vi "Zaber_Init.vi"() -> (0 "Assignment":cluster{"Microstep Size":dbl, "Device":string}[](array[cluster]), 1 "Axes Ass":bool, 2 "VISA resource name out":refnum<visa-resource-name>)   [LabVIEW 2015]
uses:
  <vilib>/Utility/file.llb/Read Delimited Spreadsheet (string).vi
  Zaber A Series/Zaber A Series.lvlib
panel:
  out "Microsteps":dbl[](array[numeric])
  out "error out":errorcluster
  out "Dev Numbers":string[](array[string])
  in  "Z":u16(ring) caption="Z (transverse)" items=["01", "02", "03"]
  in  "Y":u16(ring) caption="Y (vertical)" items=["01", "02", "03"]
  in  "X":u16(ring) caption="X (horizontal)" items=["01", "02", "03"]
  in  "Ass Axes":bool
  in  "Quit":bool
  in  "VISA resource name":refnum<visa-resource-name>
  out "Lookup file not found":bool
  in  "connect":bool
  out "Hardware Detected:":T1(array[cluster])
  out "Init Failed":bool
  # "Device Number & Axis"
  # "Model Name"
  # "Motion Type"
  # "Microstep"
  # "Assignment"
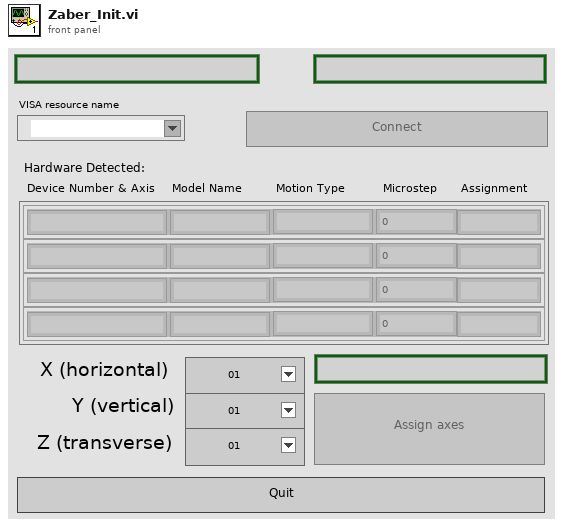
[diagram p1: front panel]
types:
  T1 = cluster{"Device Number & Axis":string, "Model Name":string, "Motion Type":string, "Microstep Size":dbl, "Assignment":string}[]
  T2 = enum8{"Enabled", "Disabled", "Disabled and Grayed Out"}
  T3 = cluster{"Device Number & Axis":string, "Model Name":string, "Motion Type":string, "Microstep Size":dbl, "Assignment":string}
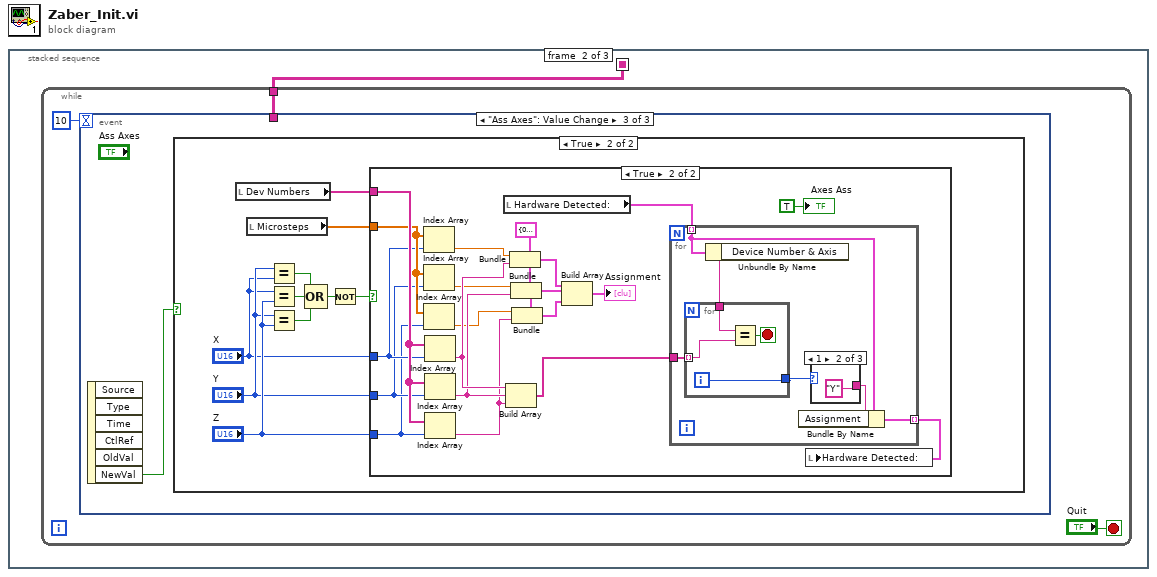
[diagram p0: block diagram]
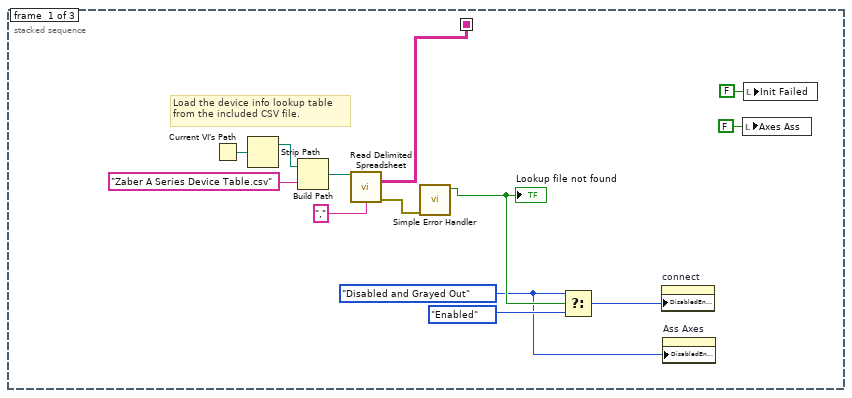
[diagram p2: hidden frame]
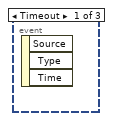
[diagram p3: hidden frame]
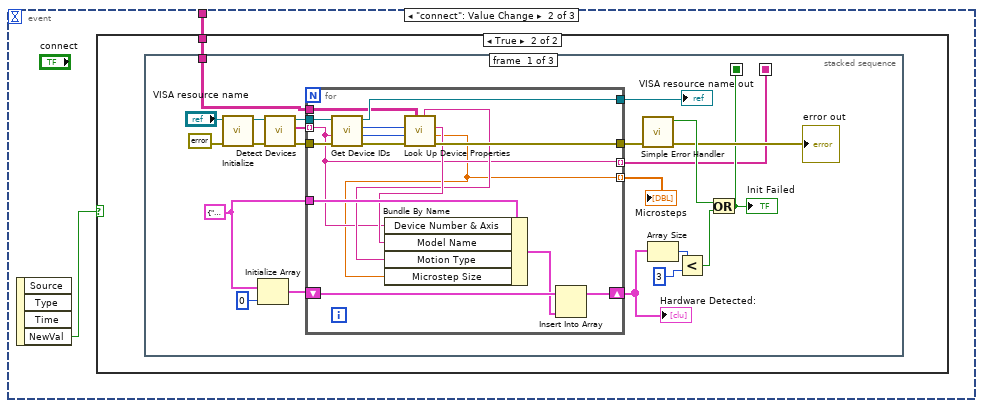
[diagram p4: hidden frame]
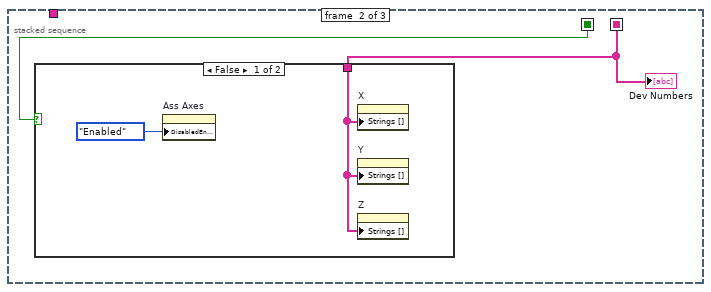
[diagram p6: hidden frame]
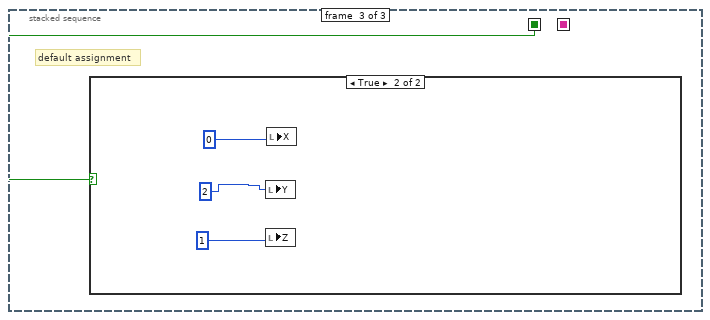
[diagram p8: hidden frame]
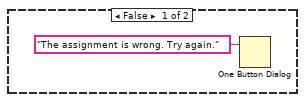
[diagram p11: hidden frame]
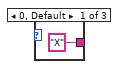
[diagram p12: hidden frame]
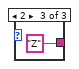
[diagram p13: hidden frame]
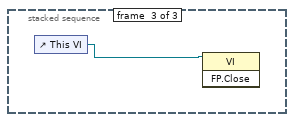
[diagram p14: hidden frame]
diagram:
  n1 = stacked-sequence {
    seq-local: [w7 _ _] -> [_ w14 _]
    frame #0 {
      w2 = T2."Disabled and Grayed Out" ("Disabled")
      # "Load the device info lookup table\nfrom the included CSV file."
      n2 = Current VI's Path() -> (path=w12:path)
      n3 = Strip Path(path=w12) -> (stripped path=w13:path)  [unwired: 1 out]
      n4 = Build Path(base path=w13, name or relative path="Zaber A Series Device Table.csv") -> (appended path=w10:path)
      n5 = call-poly <vilib>:"Read Delimited Spreadsheet.vi"("file path (dialog if empty)"=w10, "delimiter (\\t)"="," ("delimiter (\\t)")) -> ("all rows"=w7:string[][], "error out"=w8:errorcluster)  [unwired: 8 in, 4 out]
      n6 = call <vilib>:"Simple Error Handler.vi"("error in (no error)"=w8) -> ("error?"=w6:bool)  [unwired: 4 in, 4 out]
      "Lookup file not found" <- w6
      n7 = Select(t=w2, s=w6, f=T2."Enabled" ("Disabled")) -> (s? t:f=w4:T2)
      n8 = property on="connect" class="Bool (strict)"("DisabledEnum"=w4) -> ()  [unwired: 2 in, 2 out]
      n9 = property on="Ass Axes" class="Bool (strict)"("DisabledEnum"=w2) -> ()  [unwired: 2 in, 2 out]
      n10 = local write "Axes Ass"(FALSE ("Axes Ass")) -> ()
      n11 = local write "Init Failed"(FALSE ("Init Failed")) -> ()
    }
    frame #1 {
      n12 = while {
        tunnel: w14 -> [w16]
        stop <- "Quit" stop-if-true
        n13 = event shown="[2] \"Ass Axes\": Value Change" {
          selector: _ -> [_ _ _]
          dyn-events: _ -> [_ _ _]
          timeout: 10 -> [_ _ _]
          tunnel: w16 -> [_ w18 _]
          event Timeout {
            n14 = event-data() -> ()  [unwired: 1 in, 3 out]
          }
          event "connect": Value Change {
            n15 = event-data() -> ("NewVal"=w19:bool)  [unwired: 1 in, 3 out]
            n16 = case shown="True" w19 {
              tunnel: w18 -> [_ w20]
              frame False {
              }
              frame True {
                n17 = stacked-sequence {
                  seq-local: [w23 _ _] -> [_ w59 w62]
                  seq-local: [w22 _ _] -> [_ w58 _]
                  tunnel: w20 -> [w24 _ _]
                  frame #0 {
                    w29 = T3 {"Device Number & Axis"="", "Model Name"="", "Motion Type"="", "Microstep Size"=0.0, "Assignment"=""}
                    n18 = call "Initialize.vi"("error in (no error)"=errorcluster {"status"=FALSE, "code"=0, "source"=""} ("error out"), "VISA resource name"="VISA resource name") -> ("error out"=w36:errorcluster, "VISA resource name out"=w37:refnum<visa-resource-name>)  [unwired: 8 in]
                    n19 = Initialize Array(w29, 0 ("dimension size")) -> (w27:T1)
                    n20 = call "Detect Devices.vi"("error in (no error)"=w36, "VISA resource name"=w37) -> ("error out"=w39:errorcluster, "Connected Devices and Axes"=w41:string[], "VISA resource name out"=w40:refnum<visa-resource-name>)  [unwired: 6 in, 1 out]
                    n21 = for {
                      tunnel: w40 -> [w57]
                      tunnel: w39 -> [w56]
                      tunnel: [w52] -> w30
                      tunnel: w41 -> [w43] mode=indexing
                      tunnel: [w51] -> w25
                      shift-right: [w45] -> w31
                      shift-left: w27 -> [w47]
                      tunnel: w29 -> [w50]
                      tunnel: w24 -> [w44]
                      tunnel: [w43] -> w22 mode=indexing
                      tunnel: [w42] -> w21 mode=indexing
                      n22 = call "Get Device IDs.vi"("error in (no error)"=w56, "Device and Axis"=w43, "VISA resource name"=w57) -> ("error out"=w53:errorcluster, "Peripheral ID"=w54:i32, "Device ID"=w55:i32, "VISA resource name out"=w51:refnum<visa-resource-name>)  [unwired: 5 in]
                      n23 = call "Look Up Device Properties.vi"("Lookup Table"=w44, "error in (no error)"=w53, "Peripheral ID (0)"=w54, "Device ID"=w55) -> ("error out"=w52:errorcluster, "Microstep Size"=w42:dbl, "Device Name"=w49:string, "Motion Type"=w48:string)  [unwired: 4 in]
                      n24 = Bundle By Name(cluster=w50, "Device Number & Axis"=w43, "Model Name"=w49, "Motion Type"=w48, "Microstep Size"=w42) -> (w46:T3)
                      n25 = Insert Into Array(array=w47, new element=w46) -> (w45:T1)  [unwired: 1 in]
                    }
                    "Hardware Detected:" <- w31
                    "VISA resource name out" <- w25
                    "error out" <- w30
                    "Microsteps" <- w21
                    n26 = call <vilib>:"Simple Error Handler.vi"("error in (no error)"=w30) -> ("error?"=w34:bool)  [unwired: 4 in, 4 out]
                    n27 = Array Size(array=w31) -> (size(s)=w32:i32)
                    n28 = Less?(x=w32, y=3) -> (x < y?=w35:bool)
                    n29 = Or(x=w34, y=w35) -> (x .or. y?=w23:bool)
                    "Init Failed" <- w23
                  }
                  frame #1 {
                    n30 = case shown="False" w59 {
                      tunnel: w58 -> [w60 _]
                      frame False {
                        n31 = property on="Ass Axes" class="Bool (strict)"("DisabledEnum"=T2."Enabled" ("Disabled")) -> ()  [unwired: 2 in, 2 out]
                        n32 = property on="X" class="Ring (strict)"("Strings []"=w60) -> ()  [unwired: 2 in, 2 out]
                        n33 = property on="Y" class="Ring (strict)"("Strings []"=w60) -> ()  [unwired: 2 in, 2 out]
                        n34 = property on="Z" class="Ring (strict)"("Strings []"=w60) -> ()  [unwired: 2 in, 2 out]
                      }
                      frame True {
                      }
                    }
                    "Dev Numbers" <- w58
                  }
                  frame #2 {
                    # "default assignment"
                    n35 = case shown="True" w62 {
                      frame False {
                      }
                      frame True {
                        n36 = local write "Y"(2) -> ()
                        n37 = local write "Z"(1) -> ()
                        n38 = local write "X"(0) -> ()
                      }
                    }
                  }
                }
              }
            }
          }
          event "Ass Axes": Value Change {
            n39 = event-data() -> ("NewVal"=w66:bool)  [unwired: 1 in, 5 out]
            n40 = case shown="True" w66 {
              frame False {
              }
              frame True {
                n41 = local read "Dev Numbers"() -> (w71:string[])
                n42 = local read "Microsteps"() -> (w67:dbl[])
                n43 = Equal?(x="Y", y="X") -> (x = y?=w74:bool)
                n44 = Equal?(x="X", y="Z") -> (x = y?=w75:bool)
                n45 = Equal?(x="Y", y="Z") -> (x = y?=w76:bool)
                n46 = Compound Arithmetic op=OR(w74, w75, w76) -> (w73:bool)
                n47 = Not(x=w73) -> (.not. x?=w72:bool)
                n48 = case shown="True" w72 {
                  tunnel: w71 -> [_ w97]
                  tunnel: "Z" -> [_ w89]
                  tunnel: "Y" -> [_ w90]
                  tunnel: "X" -> [_ w91]
                  tunnel: w67 -> [_ w92]
                  frame False {
                    n49 = One Button Dialog(message="The assignment is wrong. Try again.") -> ()  [unwired: 1 in, 1 out]
                  }
                  frame True {
                    w84 = cluster{"Microstep Size":dbl, "Device":string} {"Microstep Size"=0.0, "Device"=""} ("cluster")
                    n50 = Index Array(array=w92, index=w91) -> (element=w88:dbl)
                    n51 = Index Array(array=w92, index=w90) -> (element=w86:dbl)
                    n52 = Index Array(array=w92, index=w89) -> (element=w83:dbl)
                    n53 = Index Array(array=w97, index=w91) -> (element=w87:string)
                    n54 = Index Array(array=w97, index=w90) -> (element=w85:string)
                    n55 = Index Array(array=w97, index=w89) -> (element=w82:string)
                    n56 = local read "Hardware Detected:"() -> (w94:T1)
                    n57 = Build Array(w87, w85, w82) -> (w95:string[])
                    n58 = Bundle(cluster=w84, "Microstep Size"=w88, "Device"=w87) -> (w81:cluster{"Microstep Size":dbl, "Device":string})
                    n59 = Bundle(cluster=w84, "Microstep Size"=w86, "Device"=w85) -> (w80:cluster{"Microstep Size":dbl, "Device":string})
                    n60 = Bundle(cluster=w84, "Microstep Size"=w83, "Device"=w82) -> (w79:cluster{"Microstep Size":dbl, "Device":string})
                    n61 = Build Array(w81, w80, w79) -> (→"Assignment":cluster{"Microstep Size":dbl, "Device":string}[])
                    n62 = for {
                      tunnel: w95 -> [w103]
                      tunnel: w94 -> [w101] mode=indexing
                      tunnel: [w100] -> w93 mode=indexing
                      n63 = Unbundle By Name(w101) -> ("Device Number & Axis"=w102:string)
                      n64 = for {
                        tunnel: w103 -> [w109] mode=indexing
                        tunnel: w102 -> [w110]
                        tunnel: [w107] -> w99
                        i -> [w107]
                        stop <- w108 stop-if-true
                        n65 = Equal?(x=w110, y=w109) -> (x = y?=w108:bool)
                      }
                      n66 = case shown="1" w99 {
                        tunnel: ["X" ("element") "Y" ("element") "Z" ("element")] -> w98
                        frame 0, Default {
                        }
                        frame 1 {
                        }
                        frame 2 {
                        }
                      }
                      n67 = Bundle By Name(cluster=w101, "Assignment"=w98) -> (w100:T3)
                    }
                    n68 = local write "Hardware Detected:"(w93) -> ()
                    "Axes Ass" <- TRUE ("Axes Ass")
                  }
                }
              }
            }
          }
        }
      }
    }
    frame #2 {
      n69 = control-ref of="This VI"() -> (w111:refnum<vi>)
      n70 = invoke class="VI" method="FP.Close"(reference=w111) -> ()  [unwired: 2 in, 3 out]
    }
  }
